vi "PUT (File).vi"(6 "timeout":i32=10000, 7 "output file":path, 8 "error in":errorcluster, 9 "file":path, 10 "url":string, 11 "http-method in":refnum<class "REST Client.lvclass">) -> (0 "error out":errorcluster, 2 "response":refnum<class "response.lvclass">, 3 "http-method out":refnum<class "REST Client.lvclass">)   [LabVIEW 2020, in "REST Client.lvlib" / "REST Client.lvclass"]
uses:
  REST Client.lvclass
  response/response.lvclass
  http-client/http-client.lvclass
  REST Client.lvclass/REST Client.ctl
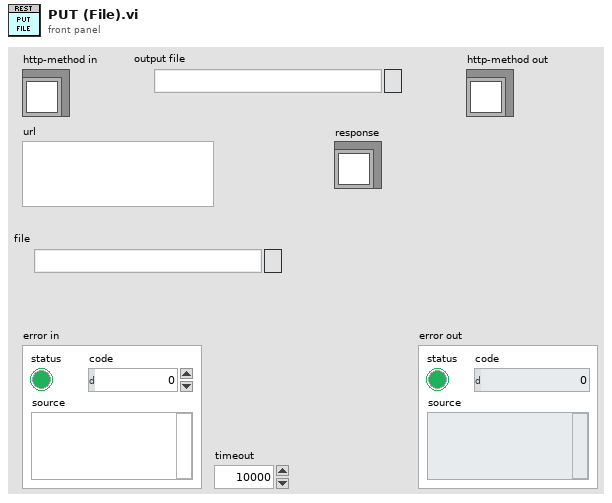
[diagram p1: front panel]
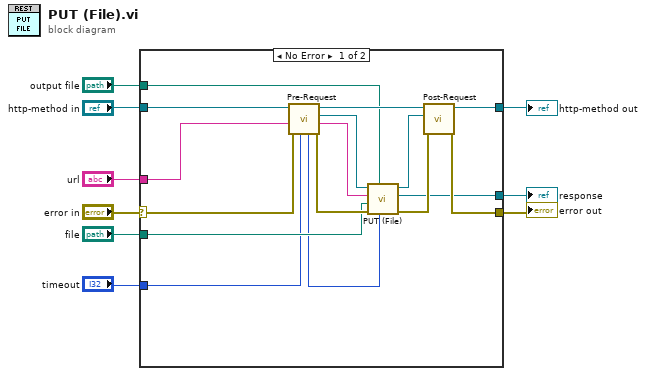
[diagram p0: block diagram]
diagram:
  n1 = case shown="No Error" "error in" {
    selector: "error in" -> [w22 w27]
    tunnel: [w19 w27] -> w1
    tunnel: [w20 w26] -> w8
    tunnel: "http-method in" -> [w21 w26]
    tunnel: "url" -> [w13 _]
    tunnel: "timeout" -> [w11 _]
    tunnel: [w18 _] -> w2
    tunnel: "output file" -> [w17 _]
    tunnel: "file" -> [w16 _]
    frame No Error {
      n2 = call "Pre-Request.vi"("timeout"=w11, "error in (no error)"=w22, "url"=w13, "REST Client in"=w21) -> ("error out"=w24:errorcluster, "Resolved URL"=w12:string, "http-client"=w15:refnum<class "http-client.lvclass">, "REST Client out"=w25:refnum<class "REST Client.lvclass">, "Timeout"=w10:i32)  [unwired: 3 in]
      n3 = call-dynamic "PUT (File).vi"("timeout"=w10, "output file"=w17, "error in"=w24, "file"=w16, "url"=w12, "http-method in"=w15) -> ("error out"=w23:errorcluster, "response"=w18:refnum<class "response.lvclass">, "http-method out"=w14:refnum<class "http-client.lvclass">)  [unwired: 3 in]
      n4 = call "Post-Request.vi"("error in (no error)"=w23, "http-method in"=w14, "REST Client in"=w25) -> ("error out"=w19:errorcluster, "REST Client out"=w20:refnum<class "REST Client.lvclass">)  [unwired: 7 in]
    }
    frame Error {
    }
  }
  "error out" <- w1
  "http-method out" <- w8
  "response" <- w2
